vi "ReadMemory 32i .vi"(8 "Error In":errorcluster, 9 "Offset":T2, 10 "Dimensions":T1={"Depth"=1, "Height"=1, "Width"=1} {"Width" min=1; "Height" min=1; "Depth" min=1}, 11 "Memory Object In":T3={"Device ID"=0, "Memeroy ID"=0, "Dimension"={"Depth"=1, "Height"=1, "Width"=1}, "Memory Type"=enum."32f"} {"Dimension"."Width" min=1; "Dimension"."Height" min=1; "Dimension"."Depth" min=1}) -> (0 "Error Out":errorcluster, 2 "Data Out":i32[][][](array[numeric]), 3 "Memory Object Out":T3={"Device ID"=0, "Memeroy ID"=0, "Dimension"={"Depth"=1, "Height"=1, "Width"=1}, "Memory Type"=enum."32f"} {"Dimension"."Width" min=1; "Dimension"."Height" min=1; "Dimension"."Depth" min=1}, 4 "ms":dbl)   [LabVIEW 2012, in "OpenCLV x64.lvlib"]
doc: "Reads i32 memory from the device to the host. This VI dynamically creates host memory based on the vector dimensions and type.\n\nIf dimension isn't provided, the entire device memory is copied to host memory."
uses:
  OpenCLV x64.lvlib
  Controls/Memory Object.ctl
  Controls/Device ID.ctl
  Controls/Memory ID.ctl
  User Controls/Array Dimensions.ctl
  Controls/Memory Type.ctl
  User Controls/Offset.ctl
  Error Checking/Add Error Functional Global.vi
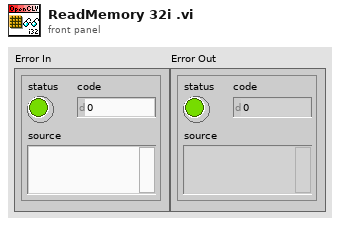
[diagram p1: front panel]
types:
  T1 = typedef "Array Dimensions.ctl" = cluster{"Depth":u64, "Height":u64, "Width":u64}
  T2 = typedef "Offset.ctl" = cluster{"X":u64, "Y":u64, "Z":u64}
  T3 = typedef "OpenCLV x64.lvlib/Memory Object.ctl" = cluster{"Device ID":T4, "Memeroy ID":T5, "Dimension":T1, "Memory Type":T6}
  T4 = typedef "OpenCLV x64.lvlib/Device ID.ctl" = u64
  T5 = typedef "OpenCLV x64.lvlib/Memory ID.ctl" = u64
  T6 = typedef "OpenCLV x64.lvlib/Memory Type.ctl" = enum16{"32f", "u8", "i8", "u16", "i16", "u32", "i32", "64f"}
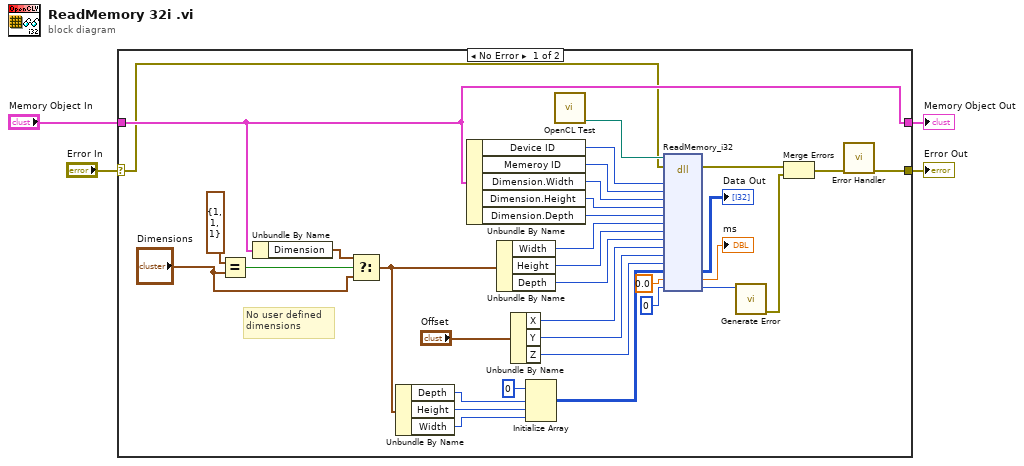
[diagram p0: block diagram]
diagram:
  n1 = case shown="No Error" "Error In" {
    selector: "Error In" -> [w5 w40]
    tunnel: [w19 w40] -> w3
    tunnel: "Memory Object In" -> [w6 w39]
    tunnel: [w6 w39] -> w1
    frame No Error {
      # "No user defined \ndimensions"
      n2 = Equal?(x=T1 {"Depth"=1, "Height"=1, "Width"=1} ("y"), y="Dimensions") -> (x = y?=w10:bool)
      n3 = Unbundle By Name(w6) -> ("Dimension"=w11:T1)
      n4 = Select(t=w11, s=w10, f="Dimensions") -> (s? t:f=w7:T1)
      n5 = Unbundle By Name(w7) -> ("Depth"=w35:u64, "Height"=w37:u64, "Width"=w38:u64)
      n6 = Unbundle By Name(w6) -> ("Device ID"=w22:T4, "Memeroy ID"=w23:T5, "Dimension.Width"=w14:u64, "Dimension.Height"=w13:u64, "Dimension.Depth"=w12:u64)
      n7 = Unbundle By Name(w7) -> ("Width"=w17:u64, "Height"=w16:u64, "Depth"=w15:u64)
      n8 = Unbundle By Name("Offset") -> ("X"=w24:u64, "Y"=w25:u64, "Z"=w26:u64)
      n9 = Initialize Array(0 ("element"), w35, w37, w38) -> (w32:i32[][][])
      n10 = call "OpenCL Test.vi"() -> ("DLL To Use"=w33:path)  [unwired: 11 in]
      n11 = dll-call lib="D:/OpenCLV/trunk/OpenCLV_x64_1.0/OpenCLV_x64.dll" fn="ReadMemory_i32"(path in=w33, error in=w5, "Labview Device"=w22, "Device Memory"=w23, "DevWidth"=w14, "DevHeight"=w13, "DevDepth"=w12, "HostWidth"=w17, "HostHeight"=w16, "HostWidth"=w15, "X Offset"=w24, "Y Offset"=w25, "Z Offset"=w26, "Data"=w32, "Time in ms"=0.0 ("Time"), "Error"=0) -> (error out=w21:errorcluster, "Data"=→"Data Out":i32[][][], "Time in ms"=→"ms":dbl, "Error"=w29:i32)  [unwired: 13 in, 1 out]
      n12 = call "Generate Error.vi"("Error"=w29) -> ("error out"=w34:errorcluster)  [unwired: 10 in]
      n13 = Merge Errors(w21, w34) -> (w20:errorcluster)
      n14 = call-poly "Error Handler.vi"("Error In"=w20) -> ("Error Out"=w19:errorcluster)  [unwired: 10 in]
    }
    frame Error {
    }
  }
  "Error Out" <- w3
  "Memory Object Out" <- w1
